vi "Compass Get Heading.vi"(0 "FPGA Information In":T2, 1 "error in (no error)":errorcluster) -> (2 "FPGA Information Out":T2, 3 "Heading (deg)":dbl, 4 "error out":errorcluster)   [LabVIEW 2012, in "Compass IO.lvlib"]
uses:
  Compass IO.lvlib
  <vilib>/IEDriver/SPIandI2C/Host/I2C/I2C Host.lvlib
  FPGA_ref.ctl
panel:
  # "Compass I2C Interface\n===\nVI to get current Heading from Compass in Degrees.\nSHOULD BE RUN @ <= 20Hz"
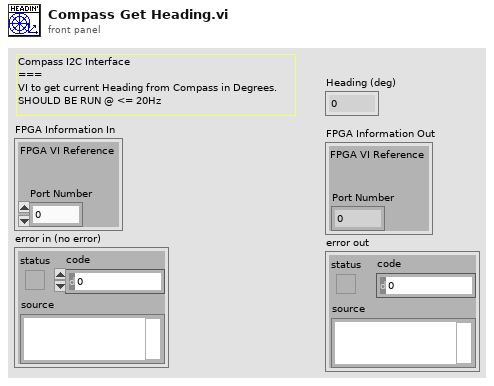
[diagram p1: front panel]
types:
  T1 = typedef "FPGA_ref.ctl" = refnum<k20>
  T2 = cluster{"FPGA VI Reference":T1, "Port Number":u8}
  T3 = cluster{"FPGA VI Reference":refnum<k20>, "Port Number":u8}
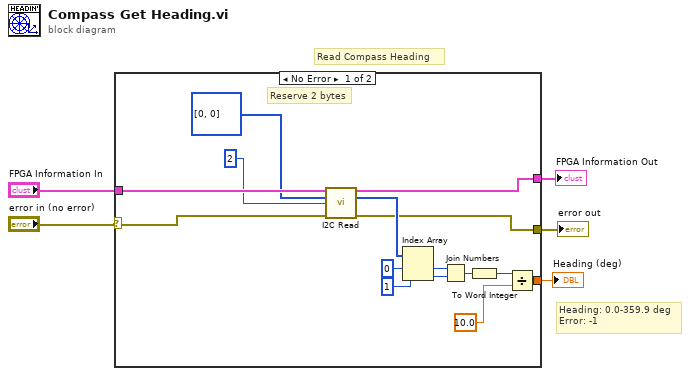
[diagram p0: block diagram]
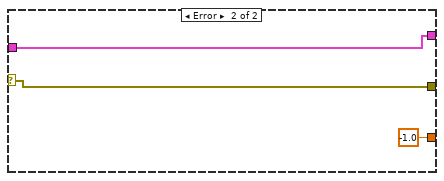
[diagram p2: hidden frame]
diagram:
  # "Heading: 0.0-359.9 deg\nError: -1"
  # "Read Compass Heading"
  n1 = case shown="No Error" "error in (no error)" {
    selector: "error in (no error)" -> [w7 w22]
    tunnel: "FPGA Information In" -> [w20 w23]
    tunnel: [w10 w23] -> w4
    tunnel: [w9 w22] -> w3
    tunnel: [w8 -1.0] -> w2
    frame No Error {
      # "Reserve 2 bytes"
      n2 = call <vilib>:"I2C Read.vi"("FPGA Information In"=w20, "Input Array"=u8[] [0, 0], "Number of Bytes to Read"=u16 2, "error in (no error)"=w7) -> ("FPGA Information Out"=w10:T3, "Data"=w11:u8[], "error out"=w9:errorcluster)  [unwired: 9 in]
      n3 = Index Array(array=w11, index #1=0 ("index"), index #2=1 ("index")) -> (element #1=w17:u8, element #2=w18:u8)
      n4 = Join Numbers(hi=w17, lo=w18) -> ((hi.lo)=w16:u16)
      n5 = To Word Integer(number=w16) -> (16bit integer=w13:i16)
      n6 = Divide(x=w13, y=10.0) -> (x/y=w8:dbl)
    }
    frame Error {
    }
  }
  "FPGA Information Out" <- w4
  "error out" <- w3
  "Heading (deg)" <- w2
